vi "Collect UI Control References.vi"(8 "Error In":errorcluster, 11 "VI Reference":refnum<vi>) -> (0 "Error Out":errorcluster, 3 "UIRefsMap":map{string, refnum<vi>}(c390))   [LabVIEW 2019, in "Utilities.lvlib"]
uses:
  Utilities.lvlib
  support/User Interface/UserInterface.lvlib
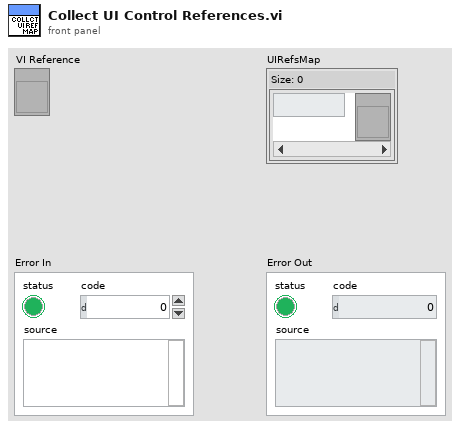
[diagram p1: front panel]
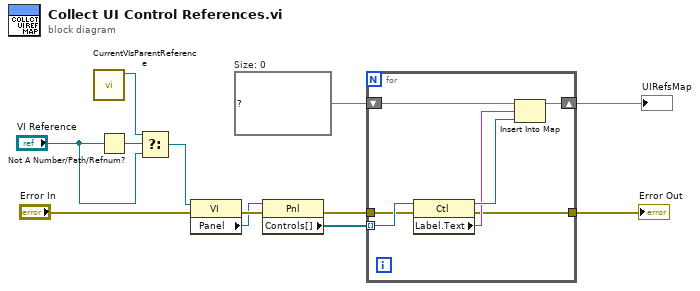
[diagram p0: block diagram]
diagram:
  w9 = map{string, refnum<vi>} {}  # Size: 0
  n1 = call "CurrentVIsParentReference.vi"() -> ("ParentVIReference"=w1:refnum<vi>)  [unwired: 11 in]
  n2 = Not A Number/Path/Refnum?(number/path/refnum="VI Reference") -> (NaN/Path/Refnum?=w4:bool)
  n3 = Select(t=w1, s=w4, f="VI Reference") -> (s? t:f=w2:refnum<vi>)
  n4 = property class="VI"(reference=w2, error in="Error In") -> (error out=w12:errorcluster, "Panel"=w11:refnum<vi>)  [unwired: 1 out]
  n5 = property class="Pnl"(reference=w11, error in=w12) -> (error out=w8:errorcluster, "Controls[]"=w10:refnum<vi>[])  [unwired: 1 out]
  n6 = for {
    tunnel: w10 -> [w18] mode=indexing
    shift-right: [w15] -> w5
    shift-left: w9 -> [w19]
    tunnel: w8 -> [w14]
    tunnel: [w13] -> w6
    n7 = property class="Ctl"(reference=w18, error in=w14) -> (reference out=w17:refnum<vi>, error out=w13:errorcluster, "Label.Text"=w16:string)
    n8 = Insert Into Map(map in=w19, key=w16, value=w17) -> (map out=w15:map{string, refnum<vi>})  [unwired: 2 out]
  }
  "Error Out" <- w6
  "UIRefsMap" <- w5
